vi "Tetra-FPGA_Boot-Success.vi"(0 "COMPORT":refnum<visa-resource-name>="COM4", 1 "Delay Time (ms)":dbl=1.0 caption="Delay Time (s)", 11 "error in (no error)":errorcluster, 12 "Command":string, 13 "Open Ser(t)":bool, 14 "Close Ser(t)":bool) -> (2 "Success":bool, 3 "output":string, 4 "comport":refnum<visa-resource-name>="COM4", 15 "error out":errorcluster)   [LabVIEW 2018]
doc: "This example performs writes and reads on a serial port, as directed by the user. You can press the Write and Read buttons, and change the Read Count, while the example is running.\n\nThe parameters set for the serial port must match the parameters of the connected instrument or device. In this example, the Read Count parameter specifies the number of bytes that the serial port reads. If there were more bytes at the port than the specified number, those bytes would not be read. If there were less bytes at the port than the specified number, you would receive a timeout error.\n\nThis example expands upon the flow control options for XON and XOFF, allowing the user to choose those control characters. Also, the user can enable or disable a termination character. Some devices require a termination character in order to identify the end of command strings. Some devices send a termination character to signify the end of data to be read. This example shows how you can end the Read operation once a termination character is detected in the buffer and/or append a termination character at the end of the Write data."
uses:
  Program Files (x86)/National Instruments/LabVIEW 2018/examples/Instrument IO/Serial/support/Serial - Settings.ctl
  Program Files (x86)/National Instruments/LabVIEW 2018/examples/Instrument IO/Serial/support/Serial - XON-XOFF Characters.ctl
  Program Files (x86)/National Instruments/LabVIEW 2018/examples/Instrument IO/Serial/support/Serial - ASCII Characters.ctl
  <vilib>/Instr/_visa.llb/VISA Flush IO Buffer Mask.ctl
  <vilib>/Utility/error.llb/DialogType.ctl
  <vilib>/Instr/_visa.llb/VISA Configure Serial Port (Instr).vi
panel:
  out "Boolean":bool
  in  "x":bool
  out "return count":u32
  in  "Max Lines to Read":i32=1000
  in  "Termination Character":u8=10 format="%.0x"
  in  "Read Count":u32=1
  in  "XON/XOFF Characters":T1={"XON"=enum."DC1", "XOFF"=enum."DC3"}
  in  "Serial Settings":T3={"baud rate"=115200, "data bits"=8, "parity"=enum."None", "stop bits"=10, "flow control"=0} {"flow control" items=["None"=0, "XON/XOFF"=1, "RTS/CTS"=2, "DTR/DSR"=4]; "stop bits" items=["1.0"=10, "1.5"=15, "2.0"=20]; "data bits" min=5 max=8 step=1; "baud rate" items=["75"=75, "110"=110, "134"=134, "150"=150, "300"=300, "600"=600, "1200"=1200, "1800"=1800, "2400"=2400, "4800"=4800, "7200"=7200, "9600"=9600, "14400"=14400, "19200"=19200, "28800"=28800, "38400"=38400, "56000"=56000, "57600"=57600, "115200"=115200, "128000"=128000, "230400"=230400]}
  # "0xA is equivalent to a '\\n' character, which is a line feed."
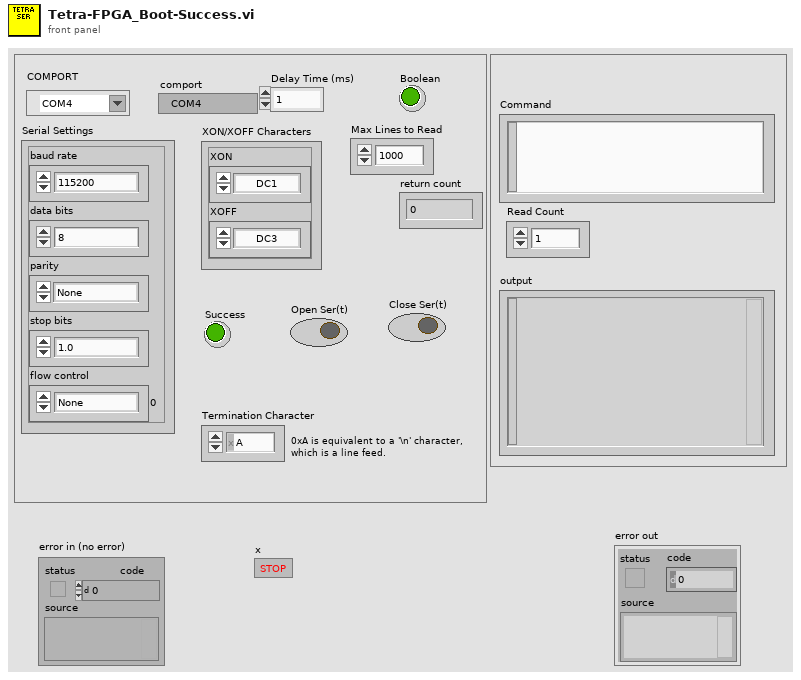
[diagram p1: front panel]
types:
  T1 = typedef "Serial - XON-XOFF Characters.ctl" = cluster{"XON":T2, "XOFF":T2}
  T2 = typedef "Serial - ASCII Characters.ctl" = enum16{"NUL", "SOH", "STX", "ETX", "EOT", "ENQ", "ACK", "BEL", "BS", "HT", "LF", "VT", "FF", "CR", "SO", "SI", "DLE", "DC1", "DC2", "DC3", "DC4", "NAK", "SYN", "ETB", "CAN", "EM", "SUB", "ESC", "FS", "GS", "RS", "US", "SP", "!", "\"", "#", "$", "%", "&", "'", "(", ")", "*", "+", ",", "- (-)", ".", "/", "0", "1", "2", "3", "4", "5", "6", "7", "8", "9", ":", ";", "<", "=", ">", "?", "@", "A", "B", "C", "D", "E", "F", "G", "H", "I", "J", "K", "L", "M", "N", "O", "P", "Q", "R", "S", "T", "U", "V", "W", "X", "Y", "Z", "[", "\\", "]", "^", "_", "`", "a", "b", "c", "d", "e", "f", "g", "h", "i", "j", "k", "l", "m", "n", "o", "p", "q", "r", "s", "t", "u", "v", "w", "x", "y", "z", "{", "|", "}", "~"}
  T3 = typedef "Serial - Settings.ctl" = cluster{"baud rate":u32, "data bits":u16, "parity":enum16{"None", "Odd", "Even", "Mark", "Space"}, "stop bits":u16, "flow control":u16}
  T4 = typedef "DialogType.ctl" = u16
  T5 = typedef "VISA Flush IO Buffer Mask.ctl" = u16
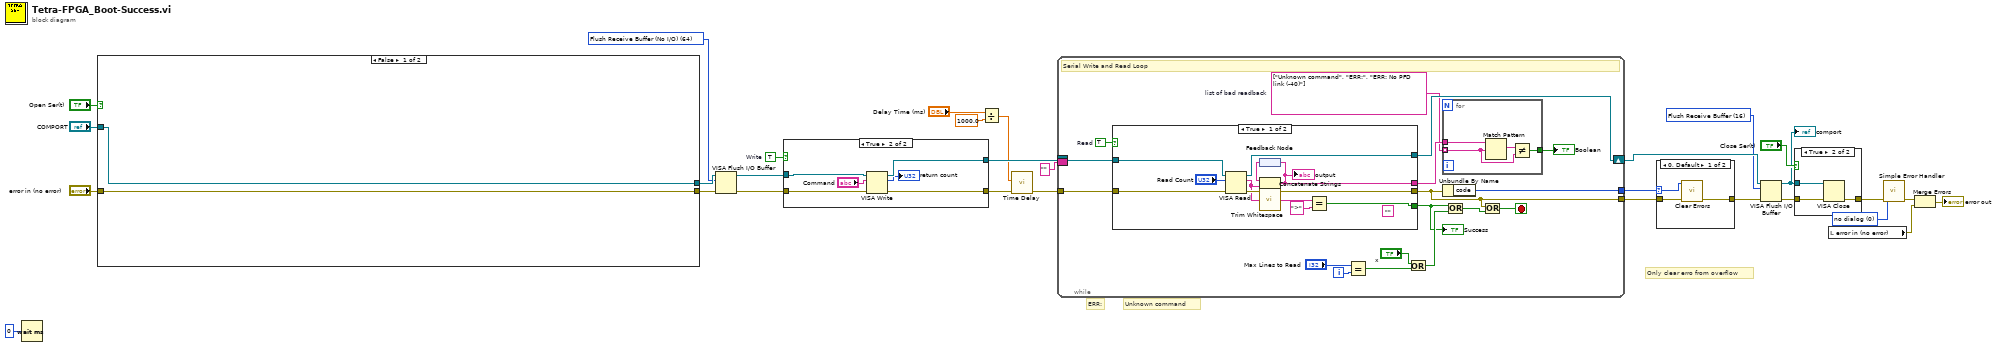
[diagram p0: block diagram]
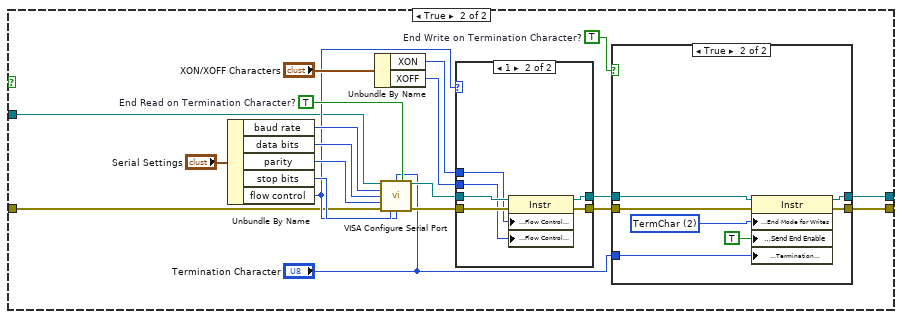
[diagram p4: hidden frame]
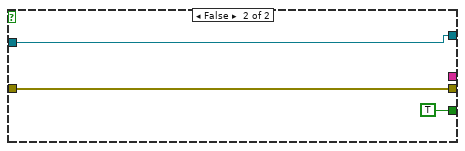
[diagram p8: hidden frame]
diagram:
  w1 = T4 0 items=["no dialog", "OK message", "continue or stop message", "OK message + warnings", "continue/stop + warnings"] ("type of dialog (OK msg:1)")
  w14 = TRUE  # Write
  w19 = T5 16 items=["Flush Receive Buffer"=16, "Write Transmit Buffer to Device"=32, "Flush Receive Buffer (No I/O)"=64, "Flush Transmit Buffer"=128] ("Mask")
  w23 = T5 64 items=["Flush Receive Buffer"=16, "Write Transmit Buffer to Device"=32, "Flush Receive Buffer (No I/O)"=64, "Flush Transmit Buffer"=128] ("Mask")
  # "Only clear erro from overflow"
  # "ERR:"
  # "Unknown command"
  n1 = Wait (ms)(milliseconds to wait=u32 0) -> ()  [unwired: 1 out]
  n2 = case shown="False" "Open Ser(t)" {
    tunnel: "COMPORT" -> [w32 w33]
    tunnel: [w31 w39] -> w28
    tunnel: [w32 w35] -> w27
    tunnel: "error in (no error)" -> [w31 w34]
    frame False {
    }
    frame True {
      w37 = TRUE  # End Write on Termination Character?
      w44 = TRUE  # End Read on Termination Character?
      n3 = Unbundle By Name("Serial Settings") -> ("baud rate"=w46:u32, "data bits"=w47:u16, "parity"=w48:enum16{"None", "Odd", "Even", "Mark", "Space"}, "stop bits"=w49:u16, "flow control"=w43:u16)
      n4 = Unbundle By Name("XON/XOFF Characters") -> ("XON"=w42:T2, "XOFF"=w41:T2)
      n5 = call-poly "VISA Configure Serial Port"("VISA resource name"=w33, "termination char\n(0xA = '\\n' = LF)"="Termination Character", "Enable Termination\nChar (T)"=w44, "baud rate (9600)"=w46, "data bits (8)"=w47, "parity (0:none)"=w48, "error in (no error)"=w34, "stop bits (10: 1 bit)"=w49, "flow control (0:none)"=w43) -> ("VISA resource name out"=w50:refnum<visa-resource-name>, "error out"=w51:errorcluster)  [unwired: 1 in, 4 out]
      n6 = case shown="1" w43 {
        tunnel: [w62 w69] -> w40
        tunnel: [w63 w68] -> w38
        tunnel: w51 -> [w62 w67]
        tunnel: w50 -> [w63 w66]
        tunnel: w42 -> [_ w65]
        tunnel: w41 -> [_ w64]
        frame Default {
        }
        frame 1 {
          n7 = property class="Instr"(reference=w66, error in=w67, "Serial Settings:Flow Control XON Character"=w65, "Serial Settings:Flow Control XOFF Character"=w64) -> (reference out=w68:refnum<visa-resource-name>, error out=w69:errorcluster)
        }
      }
      n8 = case shown="True" w37 {
        tunnel: w38 -> [w53 w61]
        tunnel: w40 -> [w54 w60]
        tunnel: [w53 w59] -> w35
        tunnel: [w54 w58] -> w39
        tunnel: "Termination Character" -> [_ w56]
        frame False {
        }
        frame True {
          w57 = u16 2 items=["None", "LastBit", "TermChar", "Break"] ("Serial Settings:Serial End Mode for Writes")
          n9 = property class="Instr"(reference=w61, error in=w60, "Serial Settings:End Mode for Writes"=w57, "Message Based Settings:Send End Enable"=TRUE, "Message Based Settings:Termination Character"=w56) -> (reference out=w59:refnum<visa-resource-name>, error out=w58:errorcluster)
        }
      }
    }
  }
  n10 = VISA Flush I/O Buffer(VISA resource name=w27, mask (16)=w23, error in (no error)=w28) -> (VISA resource name out=w17:refnum<visa-resource-name>, error out=w18:errorcluster)
  n11 = case shown="True" w14 {
    tunnel: w17 -> [w71 w76]
    tunnel: w18 -> [w70 w75]
    tunnel: [w71 w74] -> w16
    tunnel: [w70 w73] -> w6
    frame False {
    }
    frame True {
      n12 = VISA Write(VISA resource name=w76, write buffer="Command", error in (no error)=w75) -> (VISA resource name out=w74:refnum<visa-resource-name>, return count=→"return count":u32, error out=w73:errorcluster)
    }
  }
  n13 = Divide(x="Delay Time (ms)", y=1000.0) -> (x/y=w4:dbl)
  n14 = call "Time Delay"("error in (no error)"=w6, "Delay Time (s)"=w4) -> ("error out"=w5:errorcluster)  [unwired: 9 in]
  n15 = while {
    shift-right: [w94] -> w20
    shift-left: w16 -> [w86]
    tunnel: [w85] -> w13
    border: "" -> [_]
    tunnel: w5 -> [w87]
    tunnel: [w84] -> w2
    i -> [w91]
    stop <- w92 stop-if-true
    w80 = string[] ["Unknown command", "ERR:", "ERR: No PFD link (-40)"]  # list of bad readback
    w93 = TRUE  # Read
    # "Serial Write and Read Loop"
    n16 = case shown="True" w93 {
      tunnel: [w107 w112] -> w94
      tunnel: w86 -> [w109 w112]
      tunnel: [w105 w111] -> w85
      tunnel: w87 -> [w108 w111]
      tunnel: [w100 TRUE ("selection")] -> w79
      tunnel: [w99 _] -> w81
      frame True {
        (unwired) ""
        n17 = VISA Read(VISA resource name=w109, byte count="Read Count", error in (no error)=w108) -> (VISA resource name out=w107:refnum<visa-resource-name>, read buffer=w103:string, error out=w105:errorcluster)  [unwired: 1 out]
        n18 = feedback #1() -> (w104:string)
        n19 = Concatenate Strings(w104, w103) -> (w99:string)
        "output" <- w99
        n20 = feedback-in #1(w99) -> ()
        n21 = call <vilib>:"Trim Whitespace.vi"("string"=w103) -> ("trimmed string"=w102:string)  [unwired: 1 in]
        n22 = Equal?(x=w102, y=">" ("true string")) -> (x = y?=w100:bool)
      }
      frame False {
      }
    }
    "Success" <- w79
    n23 = Equal?(x="Max Lines to Read", y=w91) -> (x = y?=w88:bool)
    n24 = Or(x="x", y=w88) -> (x .or. y?=w83:bool)
    n25 = for {
      tunnel: w81 -> [w98]
      tunnel: w80 -> [w96] mode=indexing
      tunnel: [w95] -> w78
      n26 = Match Pattern(string=w98, regular expression=w96) -> (match substring=w97:string)  [unwired: 1 in, 3 out]
      n27 = Not Equal?(x=w97, y=w96) -> (x != y?=w95:bool)
    }
    "Boolean" <- w78
    n28 = Unbundle By Name(w85) -> ("code"=w84:i32)
    n29 = Or(x=w79, y=w83) -> (x .or. y?=w89:bool)
    n30 = Or(x=w85, y=w89) -> (x .or. y?=w92:bool)
  }
  n31 = case shown="0, Default" w2 {
    selector: w2 -> [w113 _]
    tunnel: w13 -> [w115 w116]
    tunnel: [w114 w116] -> w12
    frame 0, Default {
      n32 = call <vilib>:"Clear Errors.vi"("error in (no error)"=w115, "specific error code to clear (0: all)"=w113) -> ("error out"=w114:errorcluster)  [unwired: 4 in, 1 out]
    }
    frame -1073807339 {
    }
  }
  n33 = VISA Flush I/O Buffer(VISA resource name=w20, mask (16)=w19, error in (no error)=w12) -> (VISA resource name out=w11:refnum<visa-resource-name>, error out=w21:errorcluster)
  "comport" <- w11
  n34 = case shown="True" "Close Ser(t)" {
    tunnel: [w117 w120] -> w29
    tunnel: w21 -> [w117 w119]
    tunnel: w11 -> [_ w118]
    frame False {
    }
    frame True {
      n35 = VISA Close(VISA resource name=w118, error in (no error)=w119) -> (error out=w120:errorcluster)
    }
  }
  n36 = local read "error in (no error)"() -> (w8:errorcluster)
  n37 = call <vilib>:"Simple Error Handler.vi"("type of dialog (OK msg:1)"=w1, "error in (no error)"=w29) -> ("error out"=w9:errorcluster)  [unwired: 7 out]
  n38 = Merge Errors(w9, w8) -> (→"error out":errorcluster)
